vi "Init Msg Output.vi"() -> (2 "Msg Output":refnum<class "Msg Output.lvclass">)   [LabVIEW 2020, in "jettl.lvlib" / "Stopped jettl Msg.lvlib" / "Stopped Msg Output.lvlib"]
uses:
  Stopped Msg Output.lvlib
  Msg Output/Msg Output.lvclass
  Stopped Msg Output/Stopped Msg Output.lvclass
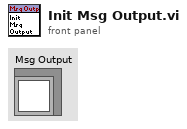
[diagram p1: front panel]
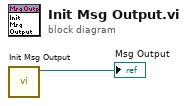
[diagram p0: block diagram]
diagram:
  n1 = call "Init Msg Output.vi"() -> ("Stopped Msg Output out"=→"Msg Output":refnum<class "Stopped Msg Output.lvclass">)  [unwired: 11 in]
